vi "Meas Proc QWTB Result Plot Panel.vi"(8 "error in":errorcluster) -> (0 "error out":errorcluster, 2 "ok?":bool, 3 "plot config":T1)   [LabVIEW 2013]
doc: "This is panel for QWTB plot configuration."
uses:
  Meas Proc QWTB Plot Scale Mode.ctl
  Meas Proc QWTB Plot Legend.ctl
  Meas Proc QWTB Plot Config.ctl
  varilib/varilib.lvlib
panel:
  in  "Show all channels":bool
  in  "btn ok":bool
  in  "Box on":bool
  in  "Grid on":bool
  in  "Show legend":T3
  in  "Y-axis style":T2
  in  "X-axis style":T2
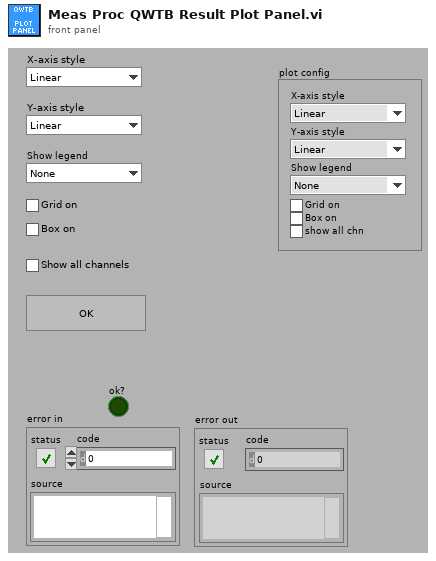
[diagram p1: front panel]
types:
  T1 = typedef "Meas Proc QWTB Plot Config.ctl" = cluster{"X-axis style":T2, "Y-axis style":T2, "Show legend":T3, "Grid on":bool, "Box on":bool, "show all chn":bool}
  T2 = typedef "Meas Proc QWTB Plot Scale Mode.ctl" = enum16{"Linear", "Log"}
  T3 = typedef "Meas Proc QWTB Plot Legend.ctl" = enum16{"None", "Best", "North", "South", "East", "West", "NorthEast", "NorthWest", "SouthEast", "SouthWest"}
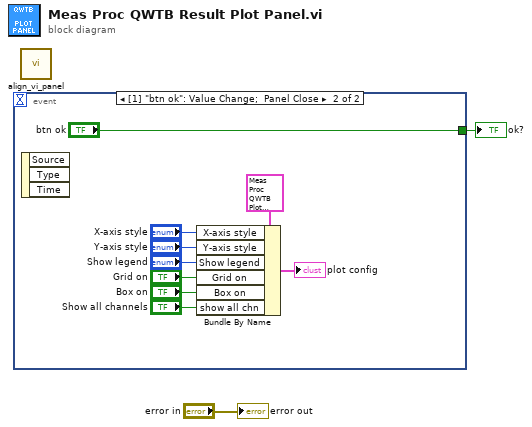
[diagram p0: block diagram]
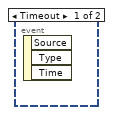
[diagram p2: hidden frame]
diagram:
  n1 = event shown="[1] \"btn ok\": Value Change;  Panel Close" {
    selector: _ -> [_ _]
    dyn-events: _ -> [_ _]
    timeout: _ -> [_ _]
    tunnel: [_ "btn ok"] -> w1
    event Timeout {
      n2 = event-data() -> ()  [unwired: 1 in, 3 out]
    }
    event "btn ok": Value Change; Panel Close {
      n3 = event-data() -> ()  [unwired: 1 in, 3 out]
      n4 = Bundle By Name(cluster=T1 {"X-axis style"=enum."Linear", "Y-axis style"=enum."Linear", "Show legend"=enum."None", "Grid on"=FALSE, "Box on"=FALSE, "show all chn"=FALSE} ("Cluster"), "X-axis style"="X-axis style", "Y-axis style"="Y-axis style", "Show legend"="Show legend", "Grid on"="Grid on", "Box on"="Box on", "show all chn"="Show all channels") -> (→"plot config":T1)
    }
  }
  "ok?" <- w1
  n5 = call "align_vi_panel.vi"() -> ()  [unwired: 11 in, 1 out]
  "error out" <- "error in"
